vi "Main IU.vi"() -> ()   [LabVIEW 2018]
uses:
  <vilib>/Analysis/baseanly.llb/Mean (DBL).vi
  <vilib>/Analysis/NI_AALBase.lvlib
panel:
  out "Gauge":dbl(knob) scale=0.0..5.0
  out "Saving Data":bool
  in  "Record Button":bool
  in  "Filename":path=path "test.lvm"
  out "Waveform Chart":waveform(dbl)[](graph)
  in  "Stop UI and RT":bool
  in  "Stop UI":bool
  in  "Setpoint":dbl
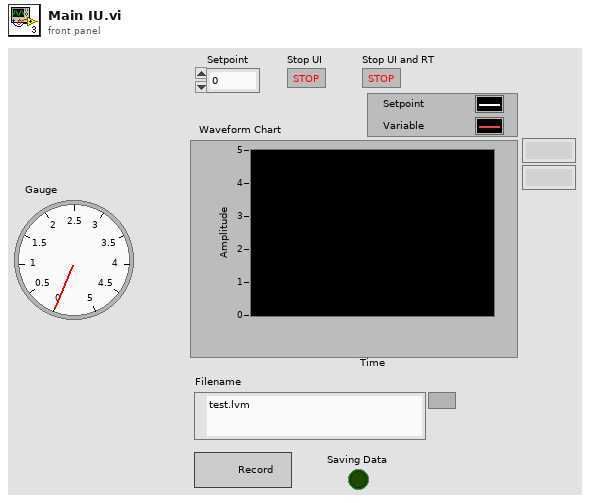
[diagram p1: front panel]
types:
  T1 = cluster{"Double":dbl, "dbl Scaled Value":dbl, "Output":dbl, "seconds since 1Jan1904":timestamp}
  T2 = cluster{"Double":dbl, "dbl Scaled Value":dbl, "Output":dbl, "seconds since 1Jan1904":timestamp}[]
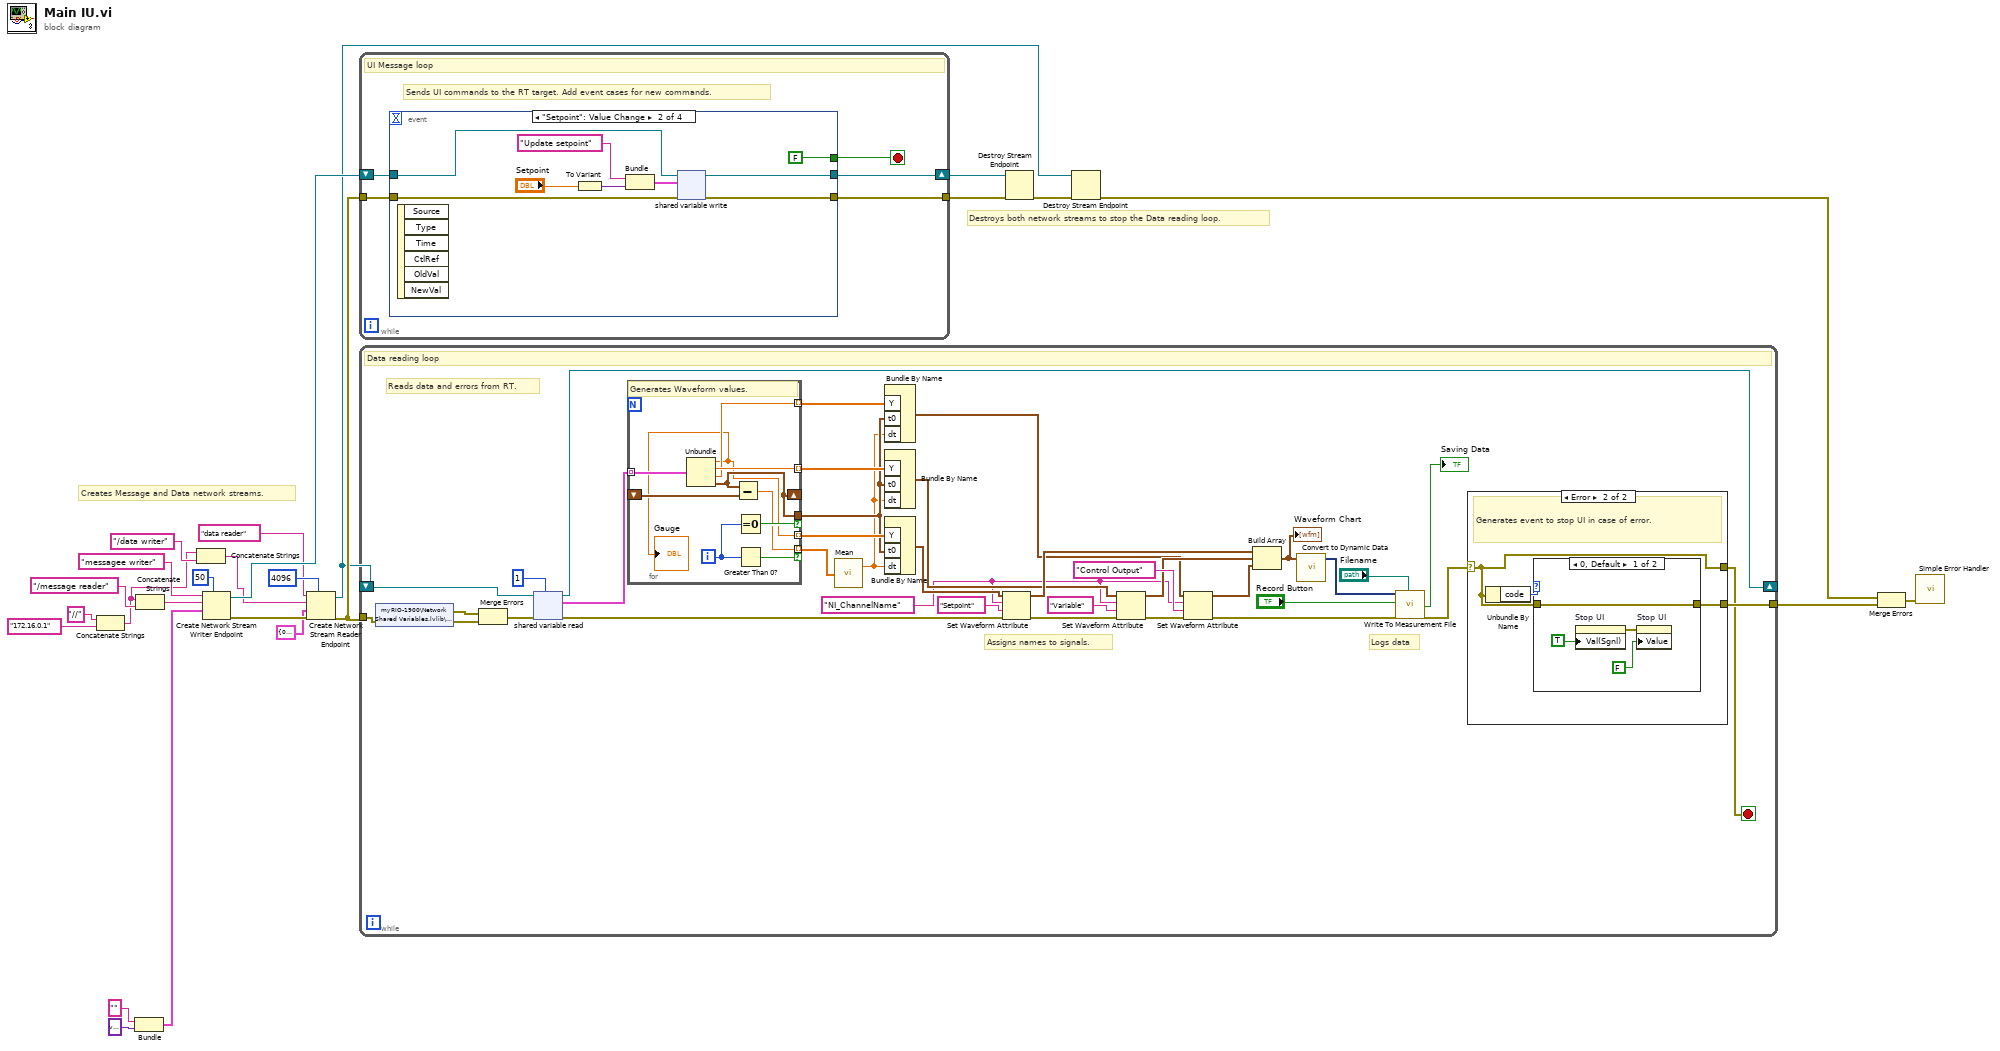
[diagram p0: block diagram]
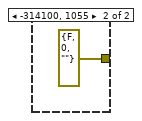
[diagram p3: hidden frame]
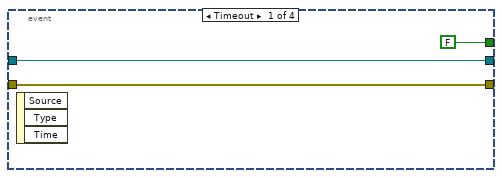
[diagram p4: hidden frame]
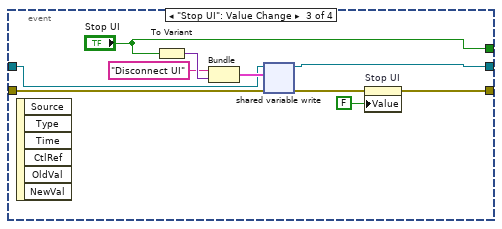
[diagram p5: hidden frame]
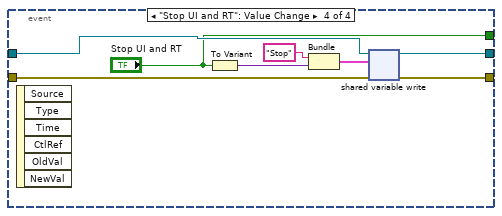
[diagram p6: hidden frame]
diagram:
  # "Destroys both network streams to stop the Data reading loop."
  # "Creates Message and Data network streams."
  n1 = Concatenate Strings("//", "172.16.0.1" ("myRIO IP")) -> (w1:string)
  n2 = Bundle("", variant) -> (w25:cluster{string, variant})  [unwired: 1 in]
  n3 = Concatenate Strings(w1, "/message reader") -> (w2:string)
  n4 = Concatenate Strings(w1, "/data writer") -> (w16:string)
  n5 = Create Network Stream Writer Endpoint(7:50 ("writer buffer size"), 9:w25, 10:w2, 11:"messagee writer" ("writer name")) -> (0:w13:errorcluster, 3:w19:refnum<k21>)  [unwired: 3 in]
  n6 = Create Network Stream Reader Endpoint(7:4096 ("reader buffer size"), 8:w13, 9:T1 {"Double"=0.0, "dbl Scaled Value"=0.0, "Output"=0.0, "seconds since 1Jan1904"=timestamp(0 s since 1904-01-01)} ("Data"), 10:w16, 11:"data reader" ("reader name")) -> (0:w12:errorcluster, 3:w5:refnum<k21>)  [unwired: 2 in]
  n7 = while {
    tunnel: w12 -> [w29]
    shift-right: [w28] -> w7
    shift-left: w19 -> [w30]
    tunnel: [w27] -> w8
    stop <- w26 stop-if-true
    # "Sends UI commands to the RT target. Add event cases for new commands."
    # "UI Message loop"
    n8 = event shown="[1] \"Setpoint\": Value Change" {
      selector: _ -> [_ _ _ _]
      dyn-events: _ -> [_ _ _ _]
      timeout: _ -> [_ _ _ _]
      tunnel: w30 -> [w33 w42 w49 w54]
      tunnel: w29 -> [w31 w41 w45 w57]
      tunnel: [w33 w36 w48 w55] -> w28
      tunnel: [w31 w35 w43 w56] -> w27
      tunnel: [FALSE ("Stop UI and RT") FALSE ("Stop UI and RT") "Stop UI" "Stop UI and RT"] -> w26
      event Timeout {
        n9 = event-data() -> ()  [unwired: 1 in, 3 out]
      }
      event "Setpoint": Value Change {
        n10 = event-data() -> ()  [unwired: 1 in, 6 out]
        n11 = To Variant(anything="Setpoint") -> (Variant=w40:variant)
        n12 = Bundle("writer name"="Update setpoint", "Variant"=w40) -> (w37:cluster{"writer name":string, "Variant":variant})  [unwired: 1 in]
        n13 = shared-variable-write(w42, w41, w37) -> (w36:refnum<k21>, w35:errorcluster)  [unwired: 1 in, 1 out]
      }
      event "Stop UI": Value Change {
        n14 = event-data() -> ()  [unwired: 1 in, 6 out]
        n15 = To Variant(anything="Stop UI") -> (Variant=w52:variant)
        n16 = Bundle("writer name"="Disconnect UI", "Variant"=w52) -> (w51:cluster{"writer name":string, "Variant":variant})  [unwired: 1 in]
        n17 = shared-variable-write(w49, w45, w51) -> (w48:refnum<k21>, w44:errorcluster)  [unwired: 1 in, 1 out]
        n18 = property on="Stop UI" class="Bool (strict)"(error in=w44, "Value"=FALSE ("Stop UI and RT")) -> (error out=w43:errorcluster)  [unwired: 1 in, 1 out]
      }
      event "Stop UI and RT": Value Change {
        n19 = event-data() -> ()  [unwired: 1 in, 6 out]
        n20 = To Variant(anything="Stop UI and RT") -> (Variant=w60:variant)
        n21 = Bundle("writer name"="Stop", "Variant"=w60) -> (w59:cluster{"writer name":string, "Variant":variant})  [unwired: 1 in]
        n22 = shared-variable-write(w54, w57, w59) -> (w55:refnum<k21>, w56:errorcluster)  [unwired: 1 in, 1 out]
      }
    }
  }
  n23 = while {
    tunnel: w12 -> [w63]
    shift-right: [w76] -> _
    shift-left: w5 -> [w96]
    tunnel: [w62] -> w9
    stop <- w61 stop-if-true
    w67 = "NI_ChannelName" ("name")
    # "Logs data"
    # "Assigns names to signals."
    # "Reads data and errors from RT."
    # "Data reading loop"
    n24 = shared-variable "myRIO-1900\\Network Shared Variables.lvlib\\error IO"(error in=w63) -> (w66:errorcluster, error out=w65:errorcluster)
    n25 = Merge Errors(w66, w65) -> (w64:errorcluster)
    n26 = shared-variable-read(w96, w64, 1 ("# elements")) -> (w76:refnum<k21>, w84:errorcluster, w94:T2)  [unwired: 1 in, 1 out]
    n27 = for {
      tunnel: w94 -> [w115] mode=indexing
      tunnel: [w106] -> w93 mode=indexing
      tunnel: [w114] -> w92 mode=indexing
      tunnel: [w113] -> w91 mode=indexing
      tunnel: [w111] -> w90 if=w112
      shift-right: [w111] -> _
      shift-left: _ -> [w110]
      tunnel: [w109] -> w68 mode=indexing if=w107
      i -> [w108]
      # "Generates Waveform values."
      n28 = Unbundle(w115) -> ("Double"=w106:dbl, "dbl Scaled Value"=w114:dbl, "Output"=w113:dbl, "seconds since 1Jan1904"=w111:timestamp)
      "Gauge" <- w106
      n29 = Subtract(x=w111, y=w110) -> (x-y=w109:dbl)
      n30 = Equal To 0?(x=w108) -> (x = 0?=w112:bool)
      n31 = Greater Than 0?(x=w108) -> (x > 0?=w107:bool)
    }
    n32 = call-poly <vilib>:"Mean.vi"("X"=w68) -> ("mean"=w89:dbl)  [unwired: 1 out]
    n33 = Bundle By Name("Y"=w91, "t0"=w90, "dt"=w89) -> (w78:waveform(dbl))  [unwired: 1 in]
    n34 = Bundle By Name("Y"=w92, "t0"=w90, "dt"=w89) -> (w79:waveform(dbl))  [unwired: 1 in]
    n35 = Bundle By Name("Y"=w93, "t0"=w90, "dt"=w89) -> (w88:waveform(dbl))  [unwired: 1 in]
    n36 = Set Waveform Attribute(4:w84, 5:"Setpoint" ("name"), 6:w67, 7:w88) -> (0:w83:errorcluster, 3:w81:waveform(dbl))  [unwired: 1 out]
    n37 = Set Waveform Attribute(4:w83, 5:"Variable" ("name"), 6:w67, 7:w79) -> (0:w82:errorcluster, 3:w80:waveform(dbl))  [unwired: 1 out]
    n38 = Set Waveform Attribute(4:w82, 5:"Control Output" ("name"), 6:w67, 7:w78) -> (0:w75:errorcluster, 3:w77:waveform(dbl))  [unwired: 1 out]
    n39 = Build Array(w81, w80, w77) -> (w74:waveform(dbl)[])
    "Waveform Chart" <- w74
    n40 = call "Convert to Dynamic Data"("Array of Waveforms"=w74) -> ("Dynamic Data Type"=w73:dynamicdata)  [unwired: 3 in]
    n41 = call "Write To Measurement File"("Signals"=w73, "Enable"="Record Button", "error in (no error)"=w75, "Filename"="Filename") -> ("Saving Data"=→"Saving Data":bool, "error out"=w69:errorcluster)  [unwired: 13 in, 1 out]
    n42 = case shown="Error" w69 {
      selector: w69 -> [w97 w98]
      tunnel: [w97 w99] -> w62
      tunnel: [w97 w98] -> w61
      frame No Error {
        # "No action required."
      }
      frame Error {
        # "Generates event to stop UI in case of error."
        n43 = Unbundle By Name(w98) -> ("code"=w100:i32)
        n44 = case shown="0, Default" w100 {
          tunnel: [w103 errorcluster {"status"=FALSE, "code"=0, "source"=""} ("error IO")] -> w99
          tunnel: w98 -> [w103 _]
          frame 0, Default {
            n45 = property on="Stop UI" class="Bool (strict)"("Val(Sgnl)"=TRUE ("Stop UI and RT")) -> (error out=w102:errorcluster)  [unwired: 2 in, 1 out]
            n46 = property on="Stop UI" class="Bool (strict)"(error in=w102, "Value"=FALSE ("Stop UI")) -> ()  [unwired: 1 in, 2 out]
          }
          frame -314100, 1055 {
          }
        }
      }
    }
  }
  n47 = Destroy Stream Endpoint(8:w8, 11:w7) -> (0:w6:errorcluster)
  n48 = Destroy Stream Endpoint(8:w6, 11:w5) -> (0:w4:errorcluster)
  n49 = Merge Errors(w4, w9) -> (w10:errorcluster)
  n50 = call <vilib>:"Simple Error Handler.vi"("error in (no error)"=w10) -> ()  [unwired: 4 in, 5 out]
